vi "MUS_winapi_midimsg_play.vi"(8 "error in":errorcluster, 9 "Stop Refnum":refnum<vi>, 10 "MUS_data":u8[](array[numeric])=array[17283 elements], 11 "Beat(Hz)":i32=140) -> (0 "error out":errorcluster)   [LabVIEW 2014]
uses:
  winmm.dll
panel:
  out "Channel":u8
  out "Note":u8
  out "Vol":u8
  out "Events":i32
  in  "stop":bool
  out "MIDI output handle":i32
  # "Events played by windows api winmm.dll MidiOutMsg\nhls"
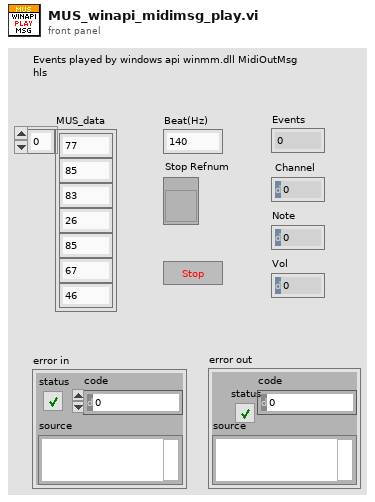
[diagram p1: front panel]
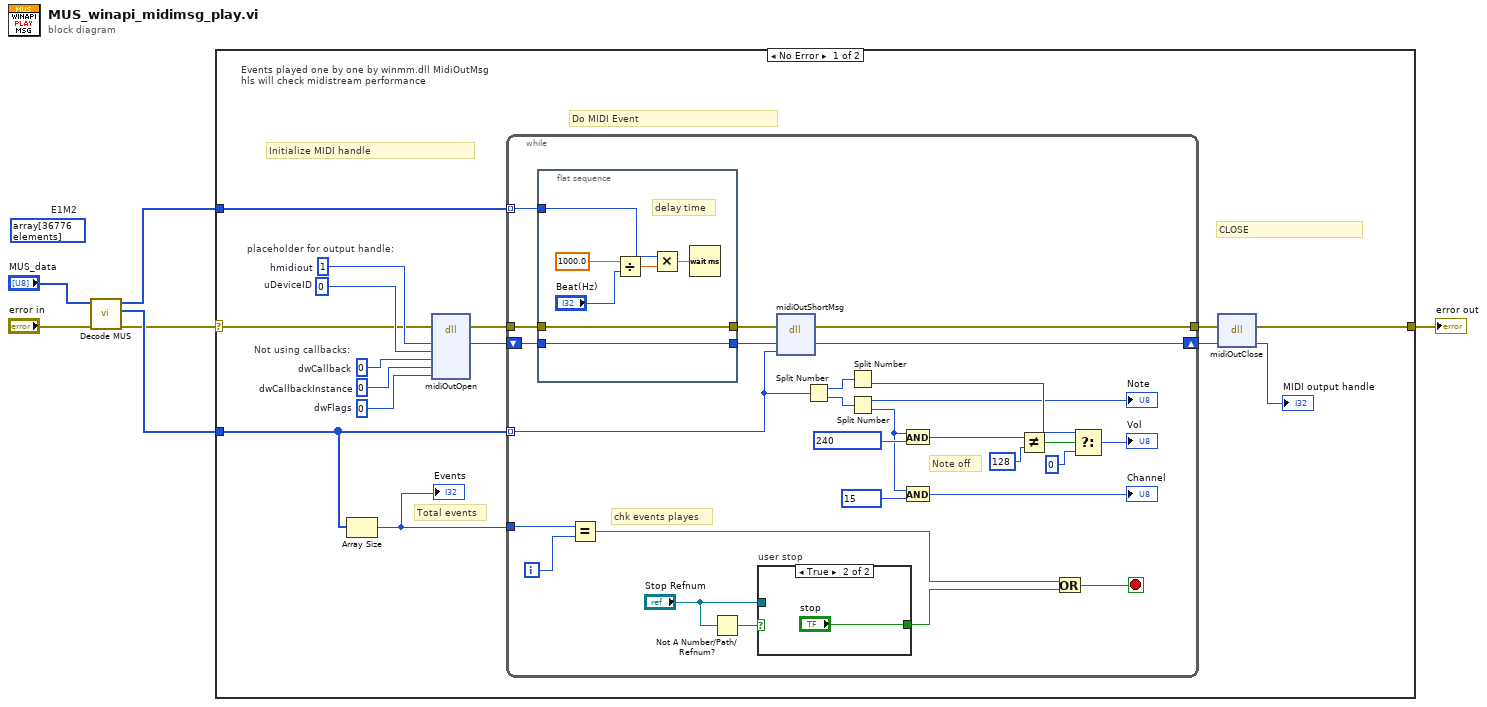
[diagram p0: block diagram]
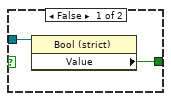
[diagram p2: hidden frame]
diagram:
  (unwired) u8[] array[36776 elements]  # E1M2
  n1 = call "Decode MUS.vi"("error in"="error in", "Music_Lump in"="MUS_data") -> ("error out"=w4:errorcluster, "midi_Msg"=w5:u32[], "delay"=w6:u32[])  [unwired: 7 in]
  n2 = case shown="No Error" w4 {
    selector: w4 -> [w10 w60]
    tunnel: w6 -> [w13 _]
    tunnel: w5 -> [w12 _]
    tunnel: [w7 w60] -> w3
    frame No Error {
      w20 = 0  # uDeviceID
      w17 = 0  # dwFlags
      w18 = 0  # dwCallbackInstance
      w19 = 0  # dwCallback
      w21 = 1  # hmidiout
      # "Events played one by one by winmm.dll MidiOutMsg\nhls will check midistream performance"
      # "Total events"
      # "Initialize MIDI handle"
      # "Do MIDI Event"
      # "CLOSE"
      # "placeholder for output handle:"
      # "Not using callbacks:"
      n3 = Array Size(array=w12) -> (size(s)=w11:i32)
      "Events" <- w11
      n4 = dll-call lib="winmm.dll" fn="midiOutOpen"(error in=w10, "hmidiout"=w21, "uDeviceID"=w20, "dwCallback"=w19, "dwCallbackInstance"=w18, "dwFlags"=w17) -> (error out=w9:errorcluster, "hmidiout"=w14:i32)  [unwired: 7 in, 1 out]
      n5 = while {
        shift-right: [w49] -> w15
        shift-left: w14 -> [w48]
        tunnel: w13 -> [w45] mode=indexing
        tunnel: w12 -> [w44] mode=indexing
        tunnel: w11 -> [w29]
        tunnel: w9 -> [w28]
        tunnel: [w26] -> w8
        i -> [w30]
        stop <- w46 stop-if-true
        # "Note off"
        # "chk events playes"
        n6 = flat-sequence {
          tunnel: w48 -> [w59]
          tunnel: [w59] -> w47
          tunnel: w45 -> [w54]
          tunnel: [w53] -> w27
          tunnel: w28 -> [w53]
          frame #0 {
            # "delay time"
            n7 = Divide(x=1000.0, y="Beat(Hz)") -> (x/y=w55:dbl)
            n8 = Multiply(x=w54, y=w55) -> (x*y=w56:dbl)
            n9 = Wait (ms)(milliseconds to wait=w56) -> ()  [unwired: 1 out]
          }
        }
        n10 = Equal?(x=w29, y=w30) -> (x = y?=w23:bool)
        n11 = Not A Number/Path/Refnum?(number/path/refnum="Stop Refnum") -> (NaN/Path/Refnum?=w25:bool)
        n12 = case "user stop" shown="True" w25 {
          tunnel: [w51 "stop"] -> w22
          tunnel: "Stop Refnum" -> [w50 _]
          frame False {
            n13 = property class="Bool (strict)"(reference=w50) -> ("Value"=w51:bool)  [unwired: 1 in, 2 out]
          }
          frame True {
          }
        }
        n14 = dll-call lib="winmm.dll" fn="midiOutShortMsg"(error in=w27, "hmidiout"=w47, "data"=w44) -> (error out=w26:errorcluster, "hmidiout"=w49:i32)  [unwired: 4 in, 1 out]
        n15 = Split Number(x=w44) -> (hi(x)=w43:u16, lo(x)=w42:u16)
        n16 = Split Number(x=w43) -> (lo(x)=w36:u8)  [unwired: 1 out]
        n17 = Split Number(x=w42) -> (hi(x)=→"Note":u8, lo(x)=w39:u8)
        n18 = And(x=w39, y=u8 240 ("f")) -> (x .and. y?=w33:u8)
        n19 = And(x=w39, y=u8 15 ("f")) -> (x .and. y?=→"Channel":u8)
        n20 = Not Equal?(x=w33, y=u8 128) -> (x != y?=w38:bool)
        n21 = Or(x=w23, y=w22) -> (x .or. y?=w46:bool)
        n22 = Select(t=w36, s=w38, f=u8 0) -> (s? t:f=→"Vol":u8)
      }
      n23 = dll-call lib="winmm.dll" fn="midiOutClose"(error in=w8, "hmidiout"=w15) -> (error out=w7:errorcluster, "hmidiout"=→"MIDI output handle":i32)  [unwired: 3 in, 1 out]
    }
    frame Error {
    }
  }
  "error out" <- w3
